vi "Input_Instrument_Positions.vi"(1 "Filepath to Save":path) -> (0 "Output string":string)   [LabVIEW 2014]
uses:
  On_Axes_Cluster.ctl
  Controls/ok_button.ctl
  File/Setup_Filetype.ctl
  Globals/Meas_global.vi
  Globals/Constants_global.vi
  Globals/Trav_pos_global.vi
panel:
  in  "On Axes":T1
  in  "OK":T2
  in  "Instrument positions when the traverse is at its origin":T3(array[cluster])=[{"Name"="", "X"=0.0, "Y"=0.0, "Z"=0.0, "Mounted On"=0, "On Axes"=enum."X Y Z"}] {"Mounted On" items=["Position N/A", "No Traverse", "A_Tunnel", "Aero_Enclosure", "Aero_Sting", "Aero_ThroughWall", "Aero_Tunnel", "Angle_Calibrator", "B_Tunnel", "D_Tunnel", "Dummy_Traverse", "EnFlo_Stack", "EnFlo_Tunnel", "EnFlo_Turntable", "Laser_Meas_Traverse", "Pitch_Yaw", "PIV_Traverse", "Tank"]; "Z" format="%#.2f"; "Y" format="%#.2f"; "X" format="%#.2f"}
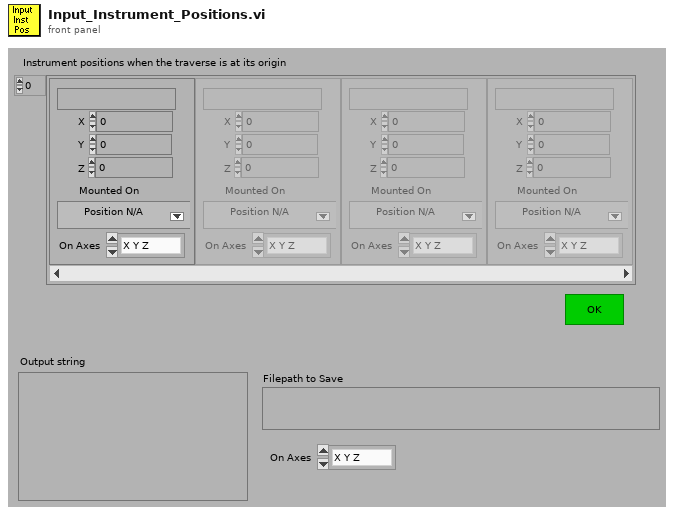
[diagram p1: front panel]
types:
  T1 = typedef "On_Axes_Cluster.ctl" = enum16{"X Y Z", "X Y", "X"}
  T2 = typedef "ok_button.ctl" = bool
  T3 = cluster{"Name":string, "X":dbl, "Y":dbl, "Z":dbl, "Mounted On":u16, "On Axes":T1}[]
  T4 = typedef "Setup_Filetype.ctl" = enum16{"Measurement Setups", "Calibration Setups", "General", "Results File Plotter Setups", "Speed Calib Tweaks"}
  T5 = typedef "Analysis_info_cluster.ctl" = cluster{"Colour":u32, "Inst type":T6, "Inst name":string, "Symbol":string, "Code name":string, "Extra Info":string, "Inst Array":T7, "Extra Titles":string[], "Extra Values":string[], "U":dbl, "u^2":dbl, "u^3":dbl, "u^4":dbl, "Skew_u":dbl, "Kurt_u":dbl, "Sd Error in Mean":dbl, "% u'/U":dbl, "X":dbl, "Y":dbl, "Z":dbl, "Timescale integral to 25%":dbl, "Sd Error in Variance":dbl, "Calib File":path, "Calib Constants":dbl[], "Output Position":bool, "Full Stats":bool, "Av Sampling Rate":dbl, "Av No of Samples":dbl, "Total Meas Time (s)":dbl, "ADAM Ch Name":string}
  T6 = typedef "Inst_type.ctl" = enum16{"Propeller anemometer", "Raw voltage", "Pressure Transducer", "Pitot-static tube", "Preston tube", "Hot wire", "Cross wire 1", "Cross wire 2", "Generic Linear", "Generic Polynomial", "Generic BackPoly", "Fast FID", "Thermocouple", "Cold wire", "Pulsed Wire", "LDA Vel", "LDA Tran time", "LDA Arr time", "Microphone"}
  T7 = typedef "Instrument_Array.ctl" = enum16{"PWA", "LDA", "Analogue"}
  T8 = cluster{"Name":string, "X":dbl, "Y":dbl, "Z":dbl, "Mounted On":u16, "On Axes":T1}
  T9 = cluster{"Values[0]":dbl, "Values[1]":dbl, "Values[2]":dbl}
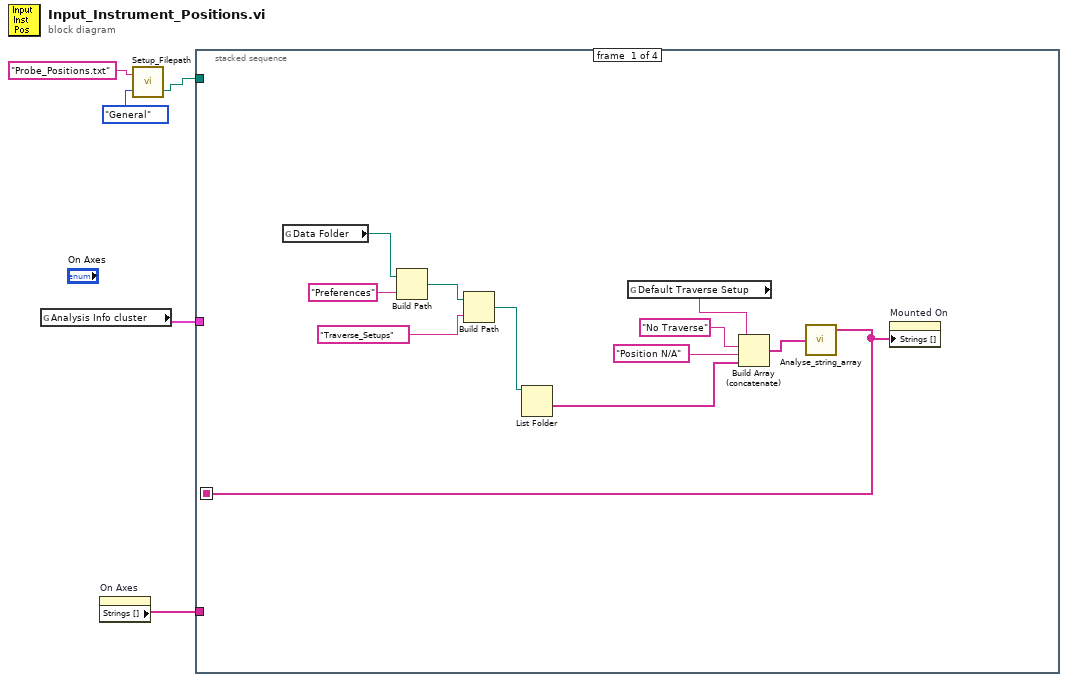
[diagram p0: block diagram]
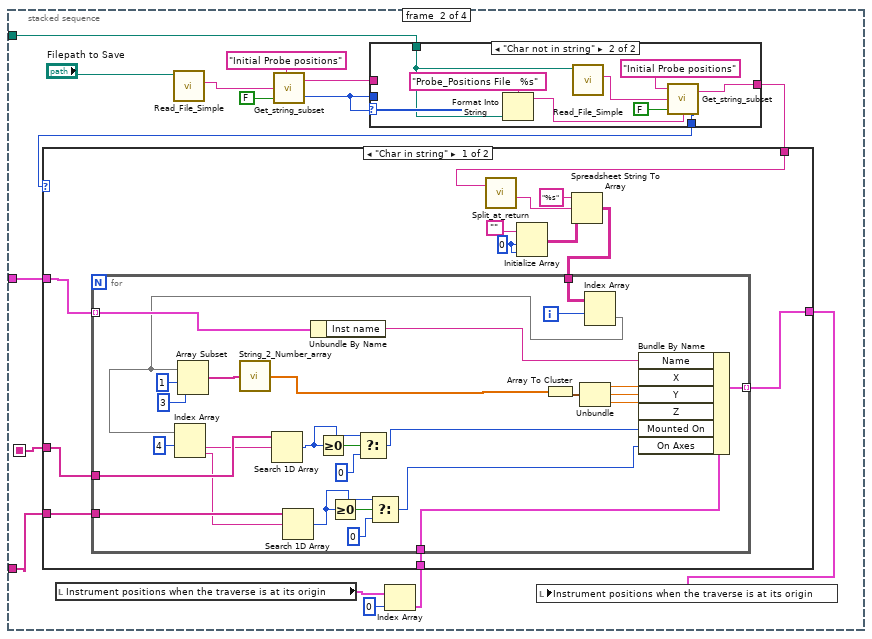
[diagram p2: hidden frame]
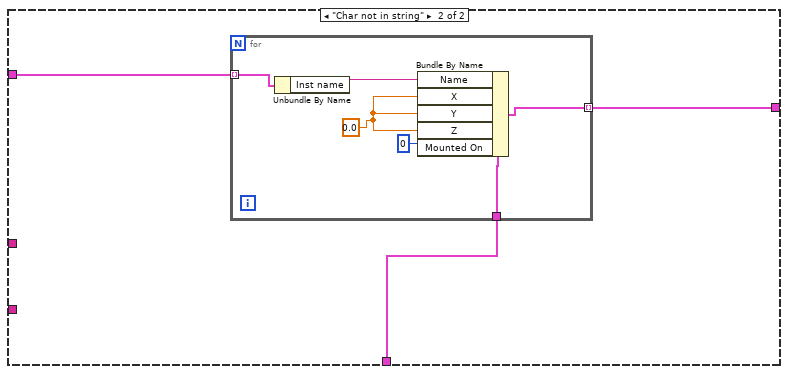
[diagram p4: hidden frame]
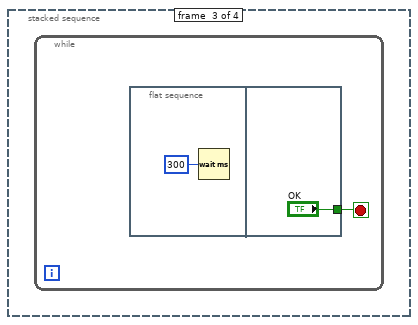
[diagram p5: hidden frame]
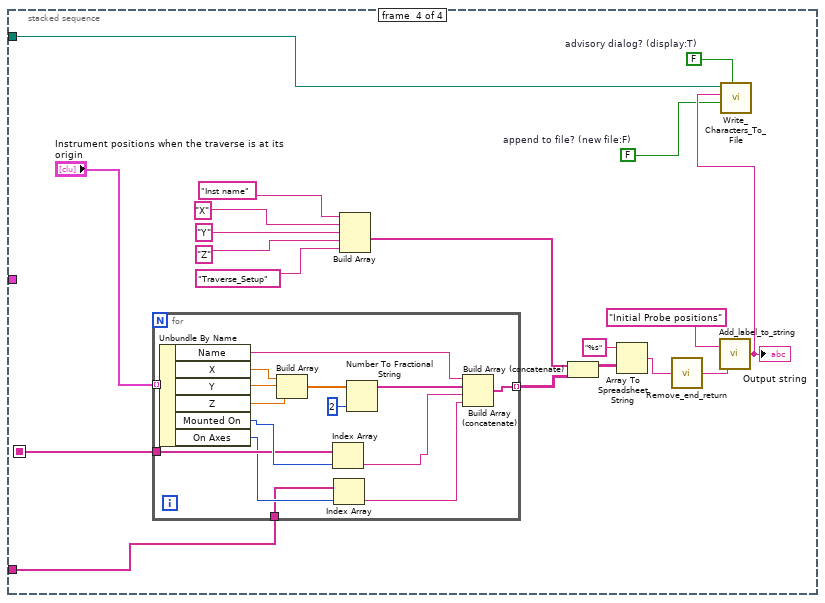
[diagram p6: hidden frame]
diagram:
  n1 = global read "Meas_global.vi" "Analysis Info cluster"() -> (w5:T5[])
  n2 = property on="On Axes" class="Enum (strict)"() -> ("Strings []"=w1:string[])  [unwired: 2 in, 2 out]
  n3 = call "Setup_Filepath.vi"("Setup File Type"=Setup_Filetype."General", "Filename in"="Probe_Positions.txt" ("name or relative path")) -> ("Filename Out"=w2:path)  [unwired: 1 out]
  n4 = stacked-sequence {
    seq-local: [w7 _ _ _] -> [_ w26 _ w100]
    tunnel: w5 -> [_ w29 _ _]
    tunnel: w2 -> [_ w20 _ w96]
    tunnel: w1 -> [_ w17 _ w95]
    frame #0 {
      n5 = global read "Constants_global.vi" "Data Folder"() -> (w13:path)
      n6 = Build Path(base path=w13, name or relative path="Preferences") -> (appended path=w15:path)
      n7 = Build Path(base path=w15, name or relative path="Traverse_Setups") -> (appended path=w12:path)
      n8 = List Folder(path=w12) -> (folder names=w9:string[])  [unwired: 1 in, 5 out]
      n9 = global read "Trav_pos_global.vi" "Default Traverse Setup"() -> (w11:string)
      n10 = Build Array (concatenate)(w11, "No Traverse" ("element"), "Position N/A" ("element"), w9) -> (w8:string[])
      n11 = call "Analyse_string_array.vi"("String array"=w8) -> ("Unique strings"=w7:string[])  [unwired: 2 out]
      n12 = property on="Mounted On" class="Ring (strict)"("Strings []"=w7) -> ()  [unwired: 2 in, 2 out]
    }
    frame #1 {
      n13 = local read "Instrument positions when the traverse is at its origin"() -> (w31:T3)
      n14 = call "Read_File_Simple.vi"("Filename"="Filepath to Save") -> ("string"=w23:string)  [unwired: 2 in, 7 out]
      n15 = call "Get_string_subset.vi"("Show Dialog?"=FALSE, "String to split"=w23, "File Label"="Initial Probe positions") -> ("Status"=w18:enum16{"Char in string", "Char not in string"}, "Output string"=w19:string)  [unwired: 1 in]
      n16 = case shown="\"Char not in string\"" w18 {
        tunnel: [w33 w39] -> w32
        tunnel: [w34 w38] -> w21
        tunnel: w20 -> [_ w36]
        tunnel: w19 -> [w34 _]
        tunnel: w18 -> [w33 _]
        frame "Char in string" {
        }
        frame "Char not in string" {
          n17 = Format Into String(format string="Probe_Positions File   %s", w36) -> (resulting string=w35:string)  [unwired: 2 in, 1 out]
          n18 = call "Read_File_Simple.vi"("Filename"=w36) -> ("string"=w40:string)  [unwired: 2 in, 7 out]
          n19 = call "Get_string_subset.vi"("String Name"=w35, "Show Dialog?"=FALSE, "String to split"=w40, "File Label"="Initial Probe positions") -> ("Status"=w39:enum16{"Char in string", "Char not in string"}, "Output string"=w38:string)
        }
      }
      n20 = Index Array(array=w31, index=0) -> (element=w28:T8)
      n21 = case shown="\"Char in string\"" w32 {
        tunnel: w29 -> [w45 w85]
        tunnel: w28 -> [w49 w84]
        tunnel: [w48 w83] -> w27
        tunnel: w26 -> [w47 _]
        tunnel: w21 -> [w46 _]
        tunnel: w17 -> [w43 _]
        frame "Char in string" {
          w51 = 0 ("Dimension Size")
          n22 = call "Split_at_return.vi"("String"=w46) -> ("after substring"=w54:string)  [unwired: 1 in, 3 out]
          n23 = Initialize Array("", w51, w51) -> (w50:string[][])
          n24 = Spreadsheet String To Array(format string="%s", spreadsheet string=w54, array type (2D Dbl)=w50) -> (array=w44:string[][])  [unwired: 1 out]
          n25 = for {
            tunnel: [w73] -> w48 mode=indexing
            tunnel: w49 -> [w72]
            tunnel: w47 -> [w71]
            tunnel: w45 -> [w64] mode=indexing
            tunnel: w44 -> [w63]
            tunnel: w43 -> [w60]
            i -> [w62]
            n26 = Unbundle By Name(w64) -> ("Inst name"=w65:string)
            n27 = Index Array(array=w63, index (row)=w62) -> (element=w61:string[])  [unwired: 1 in]
            n28 = Index Array(array=w61, index #1=4 ("index")) -> (element #1=w70:string, element #2=w59:string)  [unwired: 1 in]
            n29 = Array Subset(array=w61, index=1, length=3) -> (w80:string[])
            n30 = call "String_2_Number_array.vi"("Input String"=w80) -> ("Values"=w79:dbl[])
            n31 = Search 1D Array(1D array=w71, element=w70) -> (index of element=w68:i32)  [unwired: 1 out]
            n32 = Search 1D Array(1D array=w60, element=w59) -> (index of element=w56:i32)  [unwired: 1 out]
            n33 = Greater Or Equal To 0?(x=w68) -> (x >= 0?=w69:bool)
            n34 = Greater Or Equal To 0?(x=w56) -> (x >= 0?=w57:bool)
            n35 = Select(t=w68, s=w69, f=0) -> (s? t:f=w66:i32)
            n36 = Select(t=w56, s=w57, f=0) -> (s? t:f=w55:i32)
            n37 = Array To Cluster(array=w79) -> (cluster=w78:T9)
            n38 = Unbundle(w78) -> ("Values[0]"=w77:dbl, "Values[1]"=w76:dbl, "Values[2]"=w75:dbl)
            n39 = Bundle By Name(cluster=w72, "Name"=w65, "X"=w77, "Y"=w76, "Z"=w75, "Mounted On"=w66, "On Axes"=w55) -> (w73:T8)
          }
        }
        frame "Char not in string" {
          n40 = for {
            tunnel: w85 -> [w88] mode=indexing
            tunnel: w84 -> [w87]
            tunnel: [w86] -> w83 mode=indexing
            w89 = 0.0 ("Z")
            n41 = Unbundle By Name(w88) -> ("Inst name"=w91:string)
            n42 = Bundle By Name(cluster=w87, "Name"=w91, "X"=w89, "Y"=w89, "Z"=w89, "Mounted On"=u16 0) -> (w86:T8)
          }
        }
      }
      n43 = local write "Instrument positions when the traverse is at its origin"(w27) -> ()
    }
    frame #2 {
      n44 = while {
        stop <- w92 stop-if-true
        n45 = flat-sequence {
          tunnel: ["OK"] -> w92
          frame #0 {
            n46 = Wait (ms)(milliseconds to wait=u32 300) -> ()  [unwired: 1 out]
          }
          frame #1 {
          }
        }
      }
    }
    frame #3 {
      w97 = FALSE  # append to file? (new file:F)
      w98 = FALSE  # advisory dialog? (display:T)
      n47 = for {
        tunnel: "Instrument positions when the traverse is at its origin" -> [w128] mode=indexing
        tunnel: [w120] -> w107 mode=indexing
        tunnel: w100 -> [w118]
        tunnel: w95 -> [w115]
        n48 = Unbundle By Name(w128) -> ("Name"=w122:string, "X"=w127:dbl, "Y"=w126:dbl, "Z"=w125:dbl, "Mounted On"=w119:u16, "On Axes"=w116:T1)
        n49 = Build Array(w127, w126, w125) -> (w123:dbl[])
        n50 = Index Array(array=w118, index=w119) -> (element=w117:string)
        n51 = Index Array(array=w115, index=w116) -> (element=w114:string)
        n52 = Number To Fractional String(number=w123, precision (6)=i16 2) -> (F-format string=w121:string[])  [unwired: 2 out]
        n53 = Build Array (concatenate)(w122, w121, w117, w114) -> (w120:string[])
      }
      n54 = Build Array("Inst name", "X", "Y", "Z", "Traverse_Setup") -> (w108:string[])
      n55 = Build Array (concatenate)(w108, w107) -> (w110:string[][])
      n56 = Array To Spreadsheet String(array=w110, 3:"%s" ("format string")) -> (spreadsheet string=w112:string)  [unwired: 1 out]
      n57 = call "Remove_end_return.vi"("Input string"=w112) -> ("Output string"=w111:string)
      n58 = call "Add_label_to_string.vi"("String to write"=w111, "File Label"="Initial Probe positions") -> ("Output string"=w99:string)
      "Output string" <- w99
      n59 = call "Write_Characters_To_File.vi"("file path (dialog if empty)"=w96, "advisory dialog? (display:T)"=w98, "character string"=w99, "append to file? (new file:F)"=w97) -> ()  [unwired: 1 in, 4 out]
    }
  }
